vi "fileread.vi"() -> ()   [LabVIEW 2019]
panel:
  out "Numeric":i32
  in  "file path (use dialog)":path
  in  "access (0:read/write)":enum16{"read/write", "read-only", "write-only"}(ring)
  in  "search string/char (-) 3":string
  out "Array":string[](array[string])
  in  "search string/char (-) 2":string
  in  "search string/char (-)":string
  in  "error in":errorcluster
  out "error out":errorcluster
  out "text":string
  in  "file (use dialog)":path
  in  "prompt (Open existing file)":string
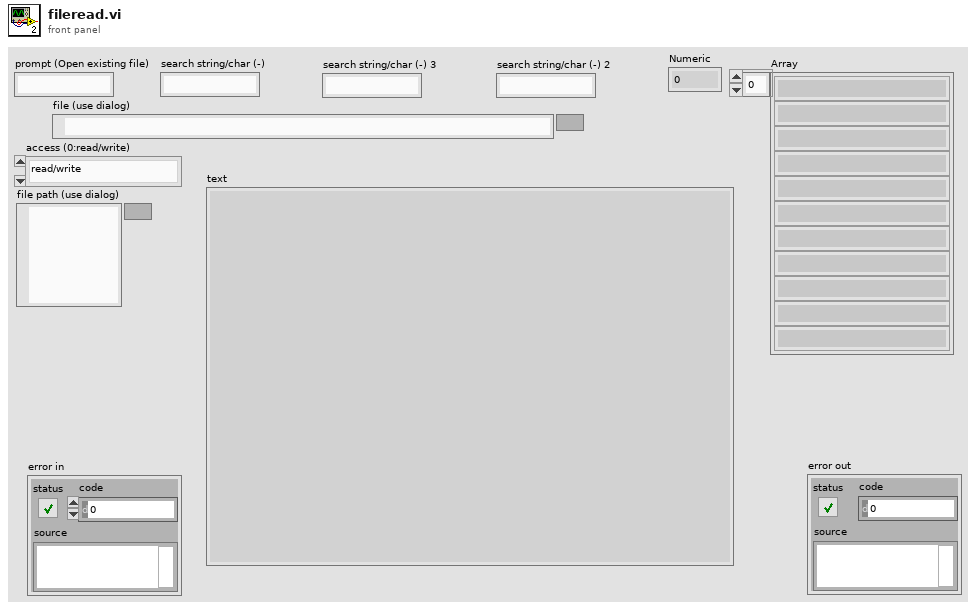
[diagram p1: front panel]
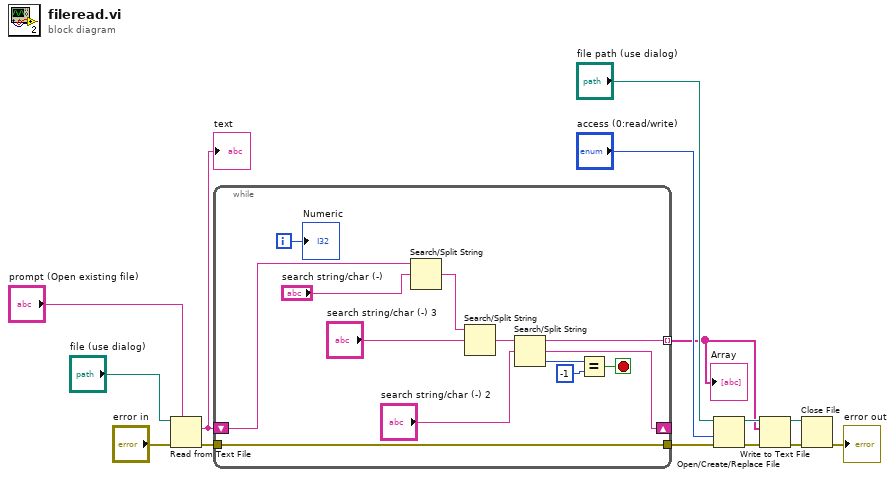
[diagram p0: block diagram]
diagram:
  n1 = Read from Text File(prompt (Open existing file)="prompt (Open existing file)", file (use dialog)="file (use dialog)", error in="error in") -> (text=w11:string, error out=w8:errorcluster)  [unwired: 1 in, 2 out]
  "text" <- w11
  n2 = while {
    shift-right: [w24] -> _
    shift-left: w11 -> [w27]
    tunnel: [w23] -> w1 mode=indexing
    tunnel: w8 -> [w16]
    tunnel: [w16] -> w7
    i -> [w15]
    stop <- w22 stop-if-true
    n3 = Search/Split String(string=w27, search string/char (-)="search string/char (-)") -> (match + rest of string=w19:string)  [unwired: 1 in, 2 out]
    n4 = Search/Split String(string=w19, search string/char (-)="search string/char (-) 3") -> (match + rest of string=w17:string)  [unwired: 1 in, 2 out]
    n5 = Search/Split String(string=w17, search string/char (-)="search string/char (-) 2") -> (substring before match=w23:string, match + rest of string=w24:string, offset of match=w21:i32)  [unwired: 1 in]
    n6 = Equal?(x=w21, y=-1) -> (x = y?=w22:bool)
    "Numeric" <- w15
  }
  "Array" <- w1
  n7 = Open/Create/Replace File(file path (use dialog)="file path (use dialog)", error in=w7, access (0:read/write)="access (0:read/write)") -> (refnum out=w5:refnum<file>, error out=w4:errorcluster)  [unwired: 3 in, 1 out]
  n8 = Write to Text File(file (use dialog)=w5, text=w1, error in=w4) -> (refnum out=w2:refnum<file>, error out=w3:errorcluster)  [unwired: 1 in, 1 out]
  n9 = Close File(refnum=w2, error in=w3) -> (error out=→"error out":errorcluster)  [unwired: 1 out]
